vi "XY Graph Get Plot & Scale Strings v2.vi"(2 "Plot Column Header":string) -> (11 "Axis Type":T1, 16 "Plot Name":string, 17 "Valid Plot Name?":bool, 18 "Scale Label":string, 19 "Valid Scale Name?":bool)   [LabVIEW 2019]
uses:
  Plot Axis Type.ctl
  <vilib>/Utility/error.llb/whitespace.ctl
panel:
  # "syntax:\nScale Label::Plot Name"
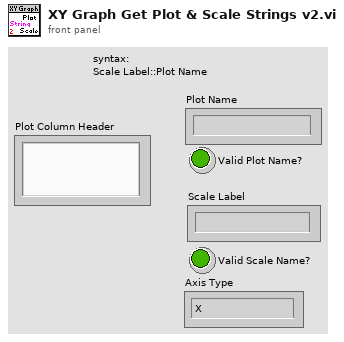
[diagram p1: front panel]
types:
  T1 = typedef "Plot Axis Type.ctl" = enum16{"X", "Y", "Z", "dX", "dY", "dZ"}
  T2 = typedef "whitespace.ctl" = u16
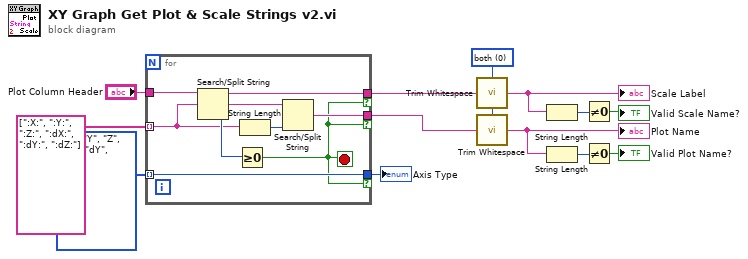
[diagram p0: block diagram]
diagram:
  w4 = T1[] [enum."X", enum."Y", enum."Z", enum."dX", enum."dY", enum."dZ"] items=["X", "Y", "Z", "dX", "dY", "dZ"]
  w12 = T2 0 items=["both", "start of string", "end of string"] ("location (both)")
  n1 = for {
    tunnel: "Plot Column Header" -> [w22]
    tunnel: string[] [":X:", ":Y:", ":Z:", ":dX:", ":dY:", ":dZ:"] ("delimiters (\\s,\\t,\\r,\\n)") -> [w17] mode=indexing
    tunnel: [w21] -> w3 if=w14
    tunnel: [w20] -> w2 if=w14
    tunnel: w4 -> [w15] mode=indexing
    tunnel: [w15] -> w1 if=w14
    stop <- w14 stop-if-true
    n2 = Search/Split String(string=w22, search string/char (-)=w17) -> (substring before match=w21:string, match + rest of string=w18:string, offset of match=w19:i32)  [unwired: 1 in]
    n3 = Greater Or Equal To 0?(x=w19) -> (x >= 0?=w14:bool)
    n4 = String Length(string=w17) -> (length=w16:i32)
    n5 = Search/Split String(string=w18, offset (0)=w16) -> (match + rest of string=w20:string)  [unwired: 1 in, 2 out]
  }
  "Axis Type" <- w1
  n6 = call <vilib>:"Trim Whitespace.vi"("string"=w3, "location (both)"=w12) -> ("trimmed string"=w7:string)
  "Scale Label" <- w7
  n7 = call <vilib>:"Trim Whitespace.vi"("string"=w2, "location (both)"=w12) -> ("trimmed string"=w11:string)
  "Plot Name" <- w11
  n8 = String Length(string=w7) -> (length=w8:i32)
  n9 = String Length(string=w11) -> (length=w10:i32)
  n10 = Not Equal To 0?(x=w8) -> (x != 0?=→"Valid Scale Name?":bool)
  n11 = Not Equal To 0?(x=w10) -> (x != 0?=→"Valid Plot Name?":bool)
